vi "THe_Machine.vi"(5 "Wait [s]":dbl, 6 "Adresse":string, 7 "error in (no error)":errorcluster, 8 "Stop Frequency":dbl, 9 "Start Frequency":dbl, 10 "Stepsize":dbl) -> (0 "error out":errorcluster, 1 "Phase Shift":cluster{dbl[], dbl[]}(graph), 2 "Error Amplitude":cluster{dbl[], dbl[]}(graph), 3 "Amplitude":cluster{dbl[], dbl[]}(graph), 4 "Error Phase Shift":cluster{dbl[], dbl[]}(graph))   [LabVIEW 2010]
uses:
  <vilib>/Utility/file.llb/Write To Spreadsheet File (DBL).vi
panel:
  out "Error Temperature":cluster{dbl[], dbl[]}(graph)
  out "Temperature":cluster{dbl[], dbl[]}(graph)
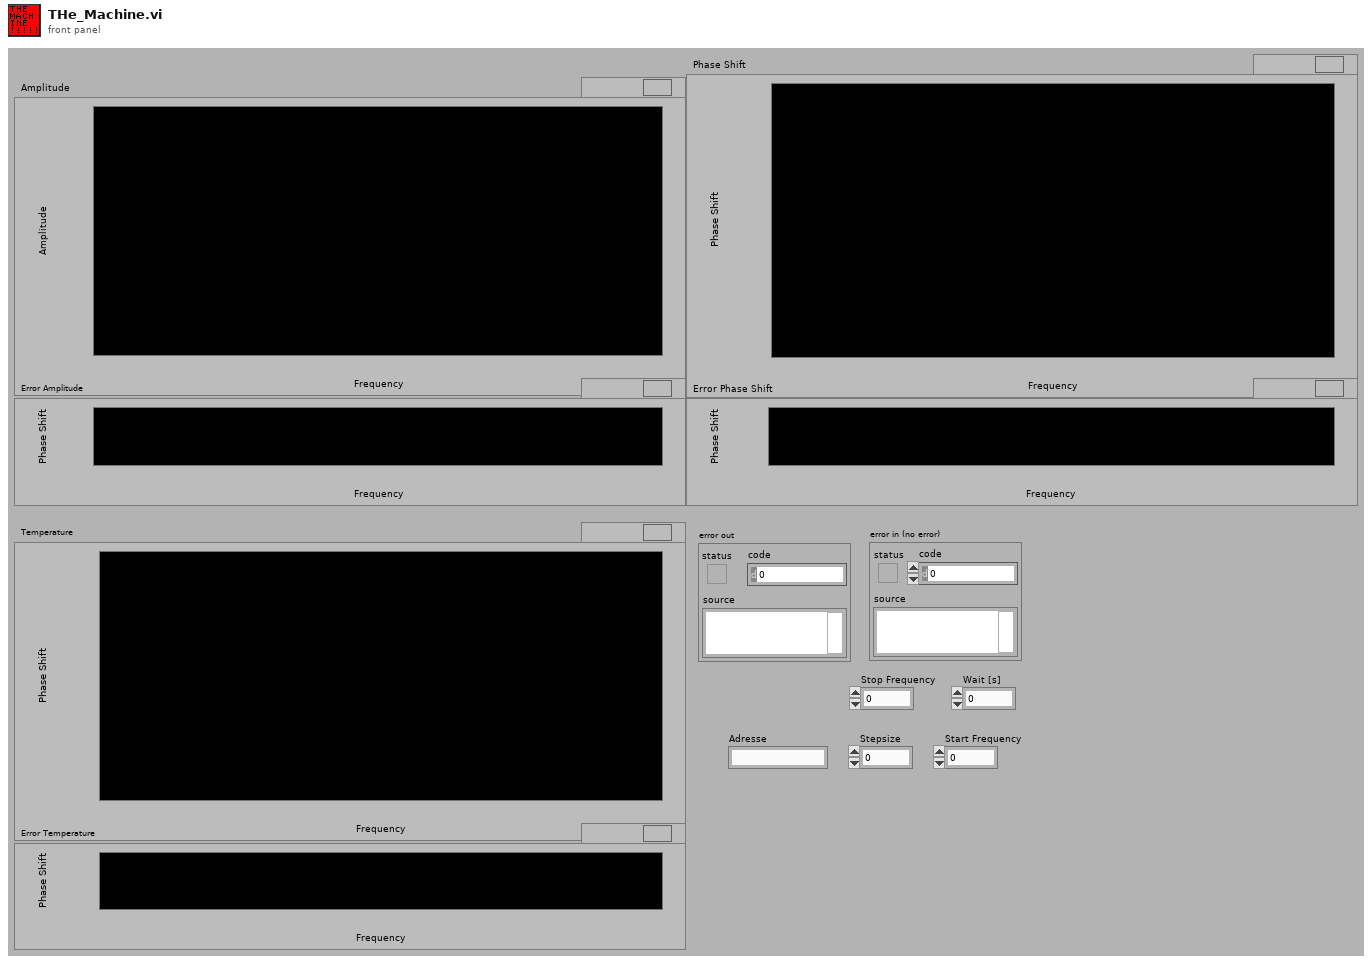
[diagram p1: front panel]
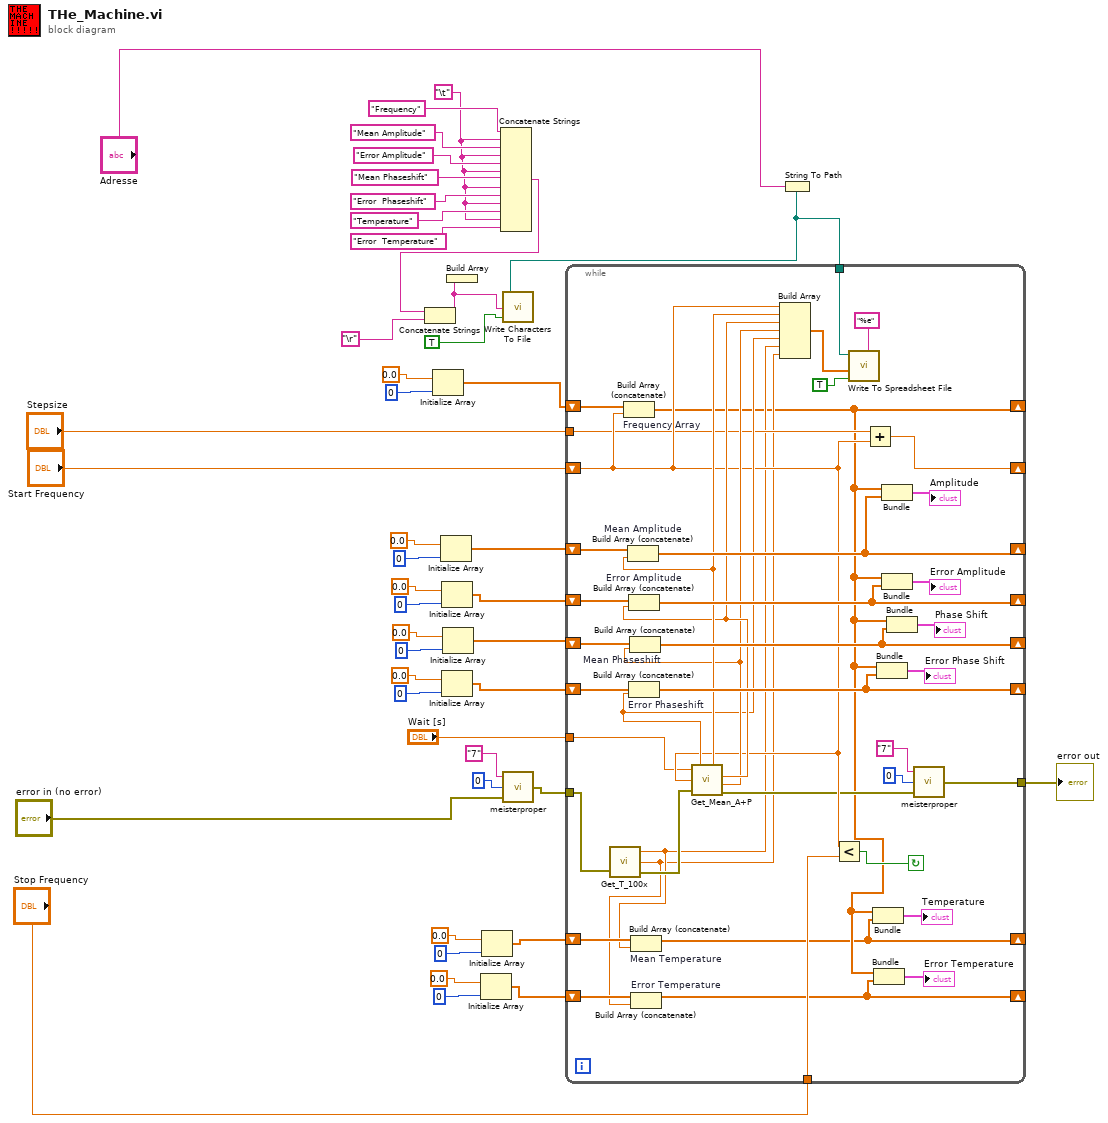
[diagram p0: block diagram]
diagram:
  w7 = "\t"
  n1 = Initialize Array(0.0, 0) -> (w41:dbl[])
  n2 = Initialize Array(0.0, 0) -> (w29:dbl[])
  n3 = Initialize Array(0.0, 0) -> (w36:dbl[])
  n4 = Initialize Array(0.0, 0) -> (w38:dbl[])
  n5 = Initialize Array(0.0, 0) -> (w37:dbl[])
  n6 = Initialize Array(0.0, 0) -> (w1:dbl[])
  n7 = Initialize Array(0.0, 0) -> (w2:dbl[])
  n8 = Concatenate Strings("Frequency", w7, "Mean Amplitude", w7, "Error Amplitude", w7, "Mean Phaseshift", w7, "Error  Phaseshift", w7, "Temperature", w7, "Error  Temperature") -> (w23:string)
  n9 = Concatenate Strings(w23, "\r") -> (w17:string)
  n10 = Build Array(w17) -> ()  [unwired: 1 out]
  n11 = call "meisterproper.vi"("error in"="error in (no error)", "mode read"=0, "adresse"="7") -> ("error out"=w26:errorcluster)
  n12 = String To Path(string="Adresse") -> (path=w44:path)
  n13 = call <vilib>:"Write Characters To File.vi"("append to file? (new file:F)"=TRUE, "character string"=w17, "file path (dialog if empty)"=w44) -> ()  [unwired: 2 in, 1 out]
  n14 = while {
    tunnel: w26 -> [w55]
    tunnel: [w59] -> w10
    tunnel: "Wait [s]" -> [w57]
    shift-right: [w86] -> _
    shift-left: "Start Frequency" -> [w63]
    tunnel: "Stepsize" -> [w62]
    tunnel: "Stop Frequency" -> [w85]
    shift-right: [w47] -> _
    shift-left: w41 -> [w81]
    shift-right: [w75] -> _
    shift-left: w29 -> [w80]
    shift-right: [w71] -> _
    shift-left: w36 -> [w79]
    shift-right: [w73] -> _
    shift-left: w37 -> [w78]
    shift-right: [w69] -> _
    shift-left: w38 -> [w77]
    tunnel: w44 -> [w56]
    shift-right: [w46] -> _
    shift-left: w2 -> [w53]
    shift-right: [w45] -> _
    shift-left: w1 -> [w52]
    stop <- w84 continue-if-true
    n15 = call "Get_T_100x.vi"("error in"=w55) -> ("error out"=w54:errorcluster, "Temperature Error"=w50:dbl, "Temperature Mean"=w51:dbl)  [unwired: 1 in]
    n16 = Build Array (concatenate) "Frequency Array"(w81, w63) -> (w47:dbl[])
    n17 = Build Array (concatenate) "Mean Temperature"(w53, w51) -> (w46:dbl[])
    n18 = Build Array (concatenate) "Error Temperature"(w52, w50) -> (w45:dbl[])
    n19 = call "Get_Mean_A+P.vi"("Wait"=w57, "Frequency"=w63, "error in (no error)"=w54) -> ("Mean Amplitude"=w68:dbl, "Error Amplitude"=w67:dbl, "Mean Phase Shift"=w66:dbl, "error out"=w58:errorcluster, "Error Phase Shift"=w65:dbl)
    n20 = Build Array (concatenate) "Mean Amplitude"(w80, w68) -> (w75:dbl[])
    n21 = Build Array (concatenate) "Error Amplitude"(w79, w67) -> (w71:dbl[])
    n22 = Build Array (concatenate) "Error Phaseshift"(w77, w65) -> (w69:dbl[])
    n23 = Build Array (concatenate) "Mean Phaseshift"(w78, w66) -> (w73:dbl[])
    n24 = Build Array(w63, w68, w67, w66, w65, w51, w50) -> (w64:dbl[])
    n25 = Less?(x=w63, y=w85) -> (x < y?=w84:bool)
    n26 = call-poly <vilib>:"Write To Spreadsheet File.vi"("format (%.3f)"="%e", "append to file? (new file:F)"=TRUE, "1D data"=w64, "file path (dialog if empty)"=w56) -> ()  [unwired: 4 in, 1 out]
    n27 = Add(x=w62, y=w63) -> (x+y=w86:dbl)
    n28 = Bundle(w47, w46) -> (→"Temperature":cluster{dbl[], dbl[]})  [unwired: 1 in]
    n29 = Bundle(w47, w45) -> (→"Error Temperature":cluster{dbl[], dbl[]})  [unwired: 1 in]
    n30 = Bundle(w47, w69) -> (→"Error Phase Shift":cluster{dbl[], dbl[]})  [unwired: 1 in]
    n31 = Bundle(w47, w75) -> (→"Amplitude":cluster{dbl[], dbl[]})  [unwired: 1 in]
    n32 = Bundle(w47, w71) -> (→"Error Amplitude":cluster{dbl[], dbl[]})  [unwired: 1 in]
    n33 = Bundle(w47, w73) -> (→"Phase Shift":cluster{dbl[], dbl[]})  [unwired: 1 in]
    n34 = call "meisterproper.vi"("error in"=w58, "mode read"=0, "adresse"="7") -> ("error out"=w59:errorcluster)
  }
  "error out" <- w10
